vi "VI Tree - file__ogtk.vi"() -> ()   [LabVIEW 2011]
uses:
  Compare Two Paths - Scalar__ogtk.vi
  Convert File Extension (Path)__ogtk.vi
  Valid Path - Traditional__ogtk.vi
  Append Path to Root if Relative - Scalar__ogtk.vi
  Strip Path Extension - Path__ogtk.vi
  File Exists - Scalar__ogtk.vi
  Build Path - Traditional__ogtk.vi
  Strip Path - Traditional__ogtk.vi
panel:
  in  "Case Constant\n(See Context Help)":bool
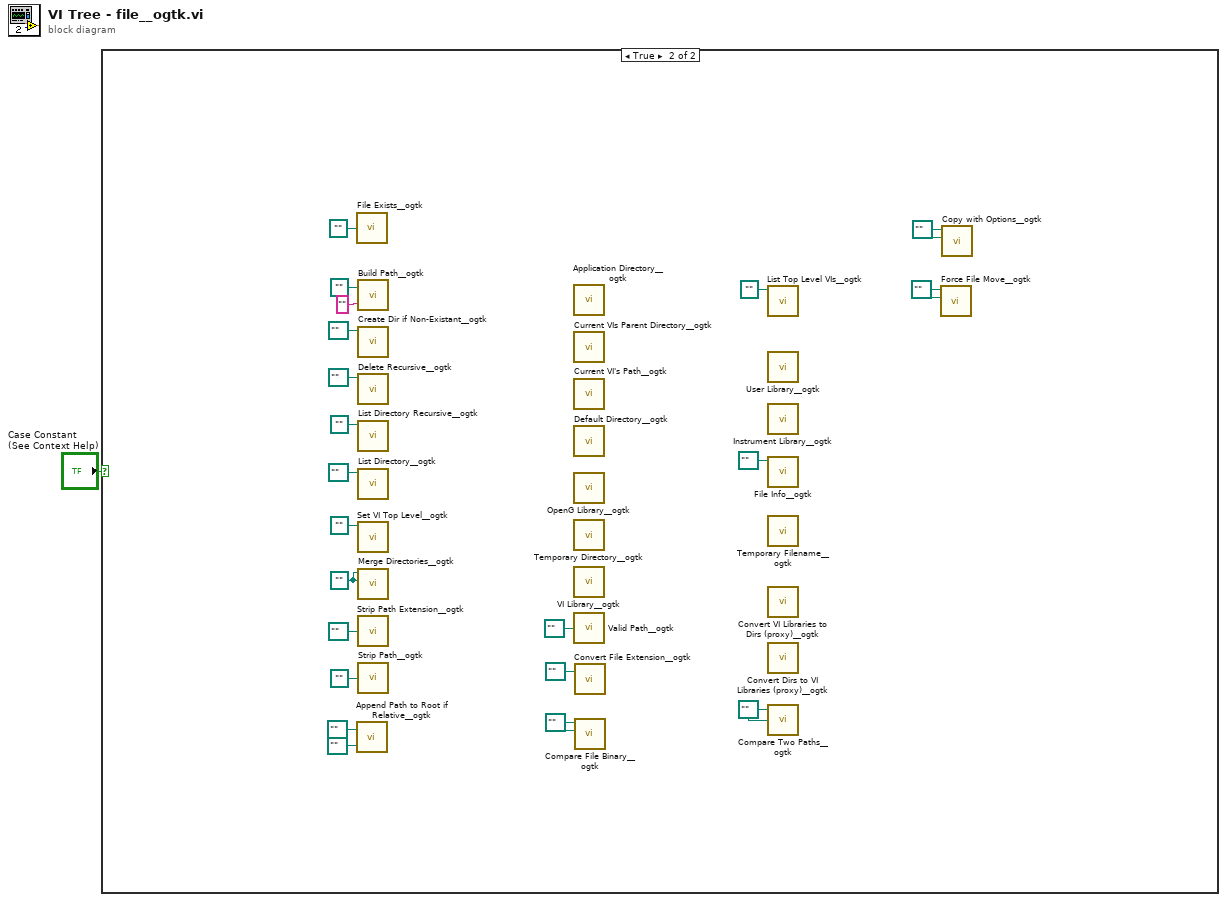
[diagram p0: block diagram]
diagram:
  n1 = case shown="True" "Case Constant\n(See Context Help)" {
    frame False {
    }
    frame True {
      w2 = path "" ("target")
      w3 = path "" ("source path")
      w4 = path "" ("path1")
      w6 = path "" ("original file")
      w19 = path "" ("target directory path")
      n2 = call-poly "File Exists__ogtk.vi"("file path"=path "") -> ()  [unwired: 6 in, 2 out]
      n3 = call-poly "Append Path to Root if Relative__ogtk.vi"("Absolute or Relative Path"=path "", "Root Path"=path "") -> ()  [unwired: 1 out]
      n4 = call-poly "Build Path__ogtk.vi"("name or relative path"="", "base path"=path "") -> ()  [unwired: 1 out]
      n5 = call "Create Dir if Non-Existant__ogtk.vi"("Directory Path"=path "") -> ()  [unwired: 8 in, 3 out]
      n6 = call "Delete Recursive__ogtk.vi"("Path"=path "") -> ()  [unwired: 9 in, 2 out]
      n7 = call "List Directory Recursive__ogtk.vi"("Path"=path "") -> ()  [unwired: 7 in, 4 out]
      n8 = call "List Directory__ogtk.vi"("directory path"=path "") -> ()  [unwired: 3 in, 4 out]
      n9 = call "Set VI Top Level__ogtk.vi"("VI Path"=path "") -> ()  [unwired: 9 in, 2 out]
      n10 = call "Merge Directories__ogtk.vi"("target directory path"=w19, "source directory path"=w19) -> ()  [unwired: 8 in, 2 out]
      n11 = call-poly "Strip Path Extension__ogtk.vi"("path"=path "") -> ()  [unwired: 2 out]
      n12 = call-poly "Strip Path__ogtk.vi"("path"=path "") -> ()  [unwired: 2 out]
      n13 = call "Application Directory__ogtk.vi"() -> ()  [unwired: 1 in, 1 out]
      n14 = call "Current VIs Parent Directory__ogtk.vi"() -> ()  [unwired: 5 in, 1 out]
      n15 = call "Current VI's Path__ogtk.vi"() -> ()  [unwired: 1 in, 1 out]
      n16 = call "Default Directory__ogtk.vi"() -> ()  [unwired: 1 in, 1 out]
      n17 = call "OpenG Library__ogtk.vi"() -> ()  [unwired: 1 in, 1 out]
      n18 = call "Temporary Directory__ogtk.vi"() -> ()  [unwired: 1 in, 1 out]
      n19 = call "VI Library__ogtk.vi"() -> ()  [unwired: 1 in, 1 out]
      n20 = call-poly "Valid Path__ogtk.vi"("path"=path "") -> ()  [unwired: 1 out]
      n21 = call-poly "Convert File Extension__ogtk.vi"("file name"=path "") -> ()  [unwired: 1 in, 2 out]
      n22 = call "Compare File Binary__ogtk.vi"("copy file"=w6, "original file"=w6) -> ()  [unwired: 4 in, 2 out]
      n23 = call "List Top Level VIs__ogtk.vi"("LLB Path"=path "") -> ()  [unwired: 8 in, 3 out]
      n24 = call "User Library__ogtk.vi"() -> ()  [unwired: 1 in, 1 out]
      n25 = call "Instrument Library__ogtk.vi"() -> ()  [unwired: 1 in, 1 out]
      n26 = call "File Info__ogtk.vi"("file"=path "") -> ()  [unwired: 5 in, 3 out]
      n27 = call "Temporary Filename__ogtk.vi"() -> ()  [unwired: 6 in, 2 out]
      n28 = call "Convert VI Libraries to Dirs (proxy)__ogtk.vi"() -> ()  [unwired: 8 in, 4 out]
      n29 = call "Convert Dirs to VI Libraries (proxy)__ogtk.vi"() -> ()  [unwired: 11 in, 1 out]
      n30 = call-poly "Compare Two Paths__ogtk.vi"("path2"=w4, "path1"=w4) -> ()  [unwired: 1 in, 3 out]
      n31 = call "Force File Move__ogtk.vi"("source"=w2, "target"=w2) -> ()  [unwired: 4 in, 2 out]
      n32 = call "Copy with Options__ogtk.vi"("target path"=w3, "source path"=w3) -> ()  [unwired: 8 in, 2 out]
    }
  }
